vi "Keller_Pop_Up.vi"(1 "data_out":dbl=1.2 step=0.01 format="%.1f", 4 "data_in":dbl format="%.2f") -> (0 "DONE":bool, 3 "Chaîne":string)   [LabVIEW 2019]
panel:
  in  "Bouton Annuler":bool
  in  "OK":bool
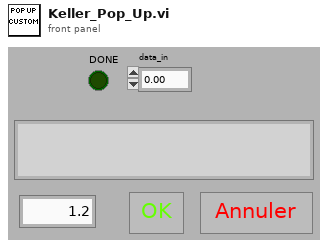
[diagram p1: front panel]
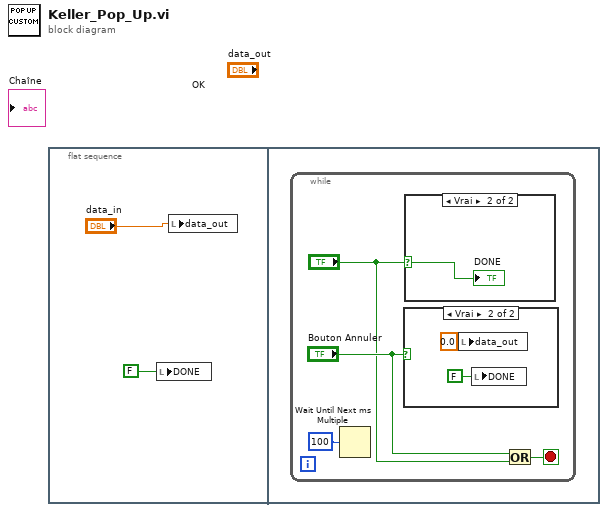
[diagram p0: block diagram]
diagram:
  n1 = flat-sequence {
    frame #0 {
      n2 = local write "DONE"(FALSE) -> ()
      n3 = local write "data_out"("data_in") -> ()
    }
    frame #1 {
      n4 = while {
        stop <- w5 stop-if-true
        n5 = Wait Until Next ms Multiple(millisecond multiple=u32 100 ("n millisecondes")) -> ()  [unwired: 1 out]
        n6 = case shown="Vrai" "Bouton Annuler" {
          frame False {
          }
          frame True {
            n7 = local write "data_out"(0.0 ("Angle")) -> ()
            n8 = local write "DONE"(FALSE ("DONE")) -> ()
          }
        }
        n9 = case shown="Vrai" "OK" {
          selector: "OK" -> [_ w9]
          frame False {
          }
          frame True {
            "DONE" <- w9
          }
        }
        n10 = Or(x="Bouton Annuler", y="OK") -> (x .or. y?=w5:bool)
      }
    }
  }
